vi "create image name.vi"(8 "error in (no error)":errorcluster, 11 "Channel in":refnum<class "SPARC4_Channel.lvclass">) -> (0 "error out":errorcluster, 3 "Channel out":refnum<class "SPARC4_Channel.lvclass">)   [LabVIEW 2018, in "SPARC4_Channel.lvclass"]
uses:
  SPARC4_Channel.lvclass
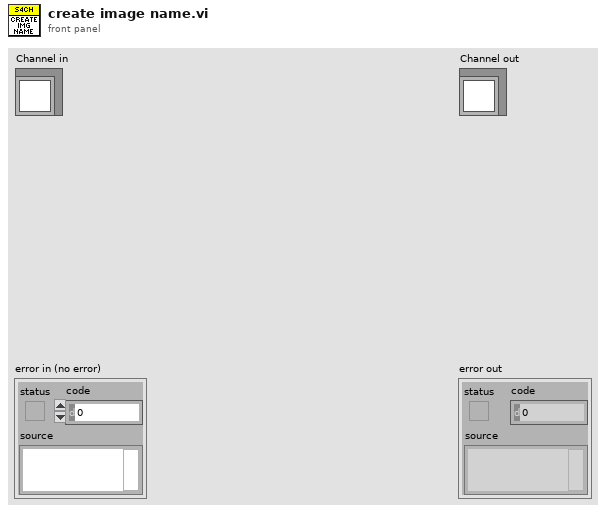
[diagram p1: front panel]
types:
  T1 = typedef "LVDateTimeRec.ctl" = cluster{"fractional second":dbl, "second":i32, "minute":i32, "hour":i32, "day of month":i32, "month":i32, "year":i32, "day of week":i32, "day of year":i32, "DST":i32}
  T2 = cluster{"Image path":path, "Channel":u8, "S4ACS mode":u16, "Log file path":path, "log level":u16}
  T3 = cluster{"CYCLES_DONE":u16, "LAST_IMAGE_NAME":string, "USED_DISK_SPACE":u16, "IMAGE_INDEX":u32, "acquisition error":bool}
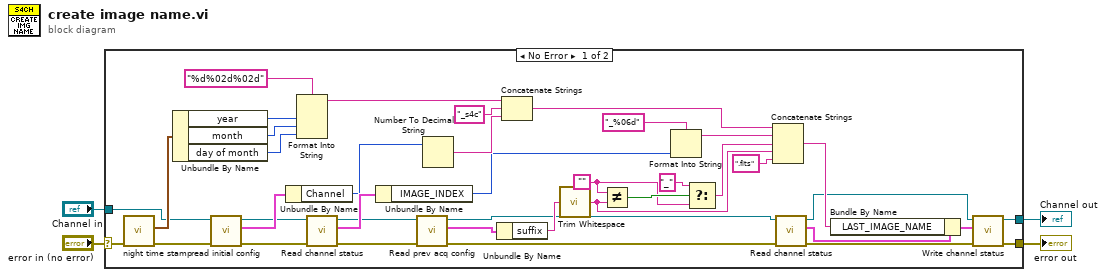
[diagram p0: block diagram]
diagram:
  n1 = case shown="No Error" "error in (no error)" {
    selector: "error in (no error)" -> [w26 w45]
    tunnel: [w20 w45] -> w3
    tunnel: [w21 w44] -> w1
    tunnel: "Channel in" -> [w12 w44]
    frame No Error {
      w34 = ""
      n2 = call "night time stamp.vi"("error in (no error)"=w26) -> ("error out"=w9:errorcluster, "date time rec"=w27:T1)  [unwired: 9 in]
      n3 = Unbundle By Name(w27) -> ("year"=w33:i32, "month"=w32:i32, "day of month"=w28:i32)
      n4 = call-dynamic "read initial config.vi"("error in (no error)"=w9, "Channel in"=w12) -> ("error out"=w8:errorcluster, "Configuration to initialize ACS"=w16:T2, "Channel out"=w11:refnum<class "SPARC4_Channel.lvclass">)  [unwired: 7 in]
      n5 = Unbundle By Name(w16) -> ("Channel"=w15:u8)
      n6 = Format Into String(format string="%d%02d%02d", w33, w32, w28) -> (resulting string=w35:string)  [unwired: 2 in, 1 out]
      n7 = call-dynamic "Read channel status.vi"("error in (no error)"=w8, "Channel in"=w11) -> ("error out"=w7:errorcluster, "channel status"=w18:T3, "Channel out"=w10:refnum<class "SPARC4_Channel.lvclass">)  [unwired: 7 in]
      n8 = Unbundle By Name(w18) -> ("IMAGE_INDEX"=w17:u32)
      n9 = call-dynamic "Read prev acq config.vi"("error in (no error)"=w7, "Channel in"=w10) -> ("error out"=w6:errorcluster, "prev acq config"=w14:cluster{"suffix":string, "#CYCLES":u32}, "Channel out"=w5:refnum<class "SPARC4_Channel.lvclass">)  [unwired: 7 in]
      n10 = Number To Decimal String(number=w15) -> (decimal integer string=w42:string)  [unwired: 1 in]
      n11 = Unbundle By Name(w14) -> ("suffix"=w13:string)
      n12 = Concatenate Strings(w35, "_s4c" ("string"), w42) -> (w41:string)
      n13 = call <vilib>:"Trim Whitespace.vi"("string"=w13) -> ("trimmed string"=w31:string)  [unwired: 1 in]
      n14 = Not Equal?(x=w34, y=w31) -> (x != y?=w40:bool)
      n15 = Format Into String(format string="_%06d", w17) -> (resulting string=w30:string)  [unwired: 2 in, 1 out]
      n16 = Select(t="_" ("string"), s=w40, f=w34) -> (s? t:f=w29:string)
      n17 = Concatenate Strings(w41, w30, w29, w31, ".fits" ("string")) -> (w24:string)
      n18 = call-dynamic "Read channel status.vi"("error in (no error)"=w6, "Channel in"=w5) -> ("error out"=w19:errorcluster, "channel status"=w25:T3, "Channel out"=w22:refnum<class "SPARC4_Channel.lvclass">)  [unwired: 7 in]
      n19 = Bundle By Name(cluster=w25, "LAST_IMAGE_NAME"=w24) -> (w23:T3)
      n20 = call-dynamic "Write channel status.vi"("error in (no error)"=w19, "channel status"=w23, "Channel in"=w22) -> ("error out"=w20:errorcluster, "Channel out"=w21:refnum<class "SPARC4_Channel.lvclass">)  [unwired: 7 in]
    }
    frame Error {
    }
  }
  "error out" <- w3
  "Channel out" <- w1
